vi "StackFromSingleWithPayload.vi"(6 "Payload":variant, 9 "Action":string) -> (1 "ActionStack out":refnum<class "Action.lvclass">[](array[class]))   [LabVIEW 2025]
uses:
  Action.lvclass
  Action.lvclass/Action.ctl
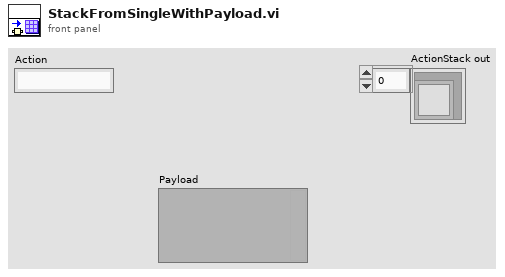
[diagram p1: front panel]
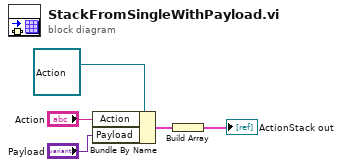
[diagram p0: block diagram]
diagram:
  n1 = Bundle By Name(cluster=refnum<class "Action.lvclass"> refnum ("ActionStack.lvclass"), "Action"="Action", "Payload"="Payload") -> (w2:cluster{})
  n2 = Build Array(w2) -> (→"ActionStack out":cluster{}[])
